vi "Set MC Analog Out.vi"(8 "error in (no error)":errorcluster, 10 "Channel":i32, 11 "Output Voltage":sgl min=-10 max=10) -> (0 "error out":errorcluster)   [LabVIEW 2016]
uses:
  Das16.llb/FromEng(single).VI
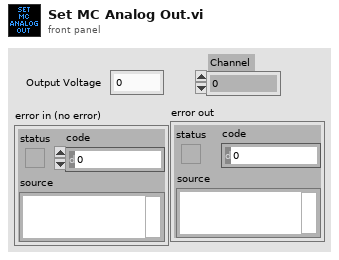
[diagram p1: front panel]
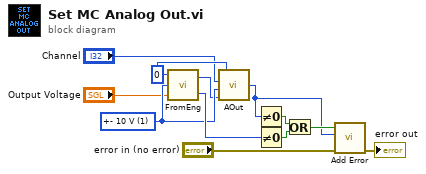
[diagram p0: block diagram]
diagram:
  w11 = 1 items=["Not Programmable"=0, "+- 20 V"=27, "+- 10 V"=1, "+- 5 V"=2, "+- 4 V"=28, "+- 2.5 V"=3, "+- 2 V"=29, "+- 1.67 V"=4, "+- 1.25 V"=5, "+- 1 V"=6, "+- .625 V"=7, "+- .5 V"=8, "+- .25 V"=30, "+- .2 V"=31, "+- .1 V"=9, "+- .05 V"=10, "+- .01 V"=11, "+- .005 V"=12, "0 - 10 V"=13, "0 - 5 V"=14, "0 - 4 V"=36, "0 - 2.5 V"=15, "0 - 2 V"=16, "0 - 1.67 V"=17, "0 - 1.25 V"=18, "0 - 1 V"=19, "0 - .5 V"=32, "0 - .25 V"=33, "0 - .2 V"=34, "0 - .1 V"=20, "0 - .02 V"=35, "0 - .01 V"=21, "4 - 20 mA"=22, "2 - 10 mA"=23, "1 - 5 mA"=24, ".5 - 2.5 mA"=25, "0 - 20 mA"=26] ("Range")
  w9 = u32 0 ("BoardNum (0)")
  n1 = call-poly "FromEng.VI"("Eng Units"="Output Voltage", "Range"=w11, "BoardNum (0)"=w9) -> ("ErrCode"=w12:i32, "DA Data"=w10:u16)
  n2 = call "AOut.VI"("DataValue"=w10, "Range"=w11, "Channel"="Channel", "BoardNum"=w9) -> ("ErrCode"=w2:i32)
  n3 = Not Equal To 0?(x=w2) -> (x != 0?=w8:bool)
  n4 = Not Equal To 0?(x=w12) -> (x != 0?=w7:bool)
  n5 = Or(x=w8, y=w7) -> (x .or. y?=w6:bool)
  n6 = call "Add Error.vi"("error in (no error)"="error in (no error)", "error code (0)"=w2, "error?"=w6) -> ("error out"=→"error out":errorcluster)  [unwired: 8 in]
